vi "Initialize.vi"(8 "error in":errorcluster, 11 "Plugin in":refnum<class "DateTimeChannel.lvclass">) -> (0 "error out":errorcluster, 3 "Plugin out":refnum<class "DateTimeChannel.lvclass">)   [LabVIEW 2023, in "DateTimeChannel.lvlib" / "DateTimeChannel.lvclass"]
uses:
  DateTimeChannel.lvclass
  C:/Program Files/National Instruments/LabVIEW 2023/vi.lib/FlexLogger/SDK/PluginSDK.lvlibp/PEFClasses/SDK/Plugin/Plugin.lvclass
  <vilib>/FlexLogger/SDK/PluginSDK.lvlibp/PEFClasses/SDK/Processing Element/Timing Parameters.ctl
  <vilib>/FlexLogger/SDK/PluginSDK.lvlibp/PEFClasses/SDK/Processing Element/Timing Method.ctl
  <vilib>/FlexLogger/SDK/PluginSDK.lvlibp/PEFClasses/SDK/Channel/Data Type_v2.ctl
  <vilib>/FlexLogger/SDK/PluginSDK.lvlibp/PEFClasses/SDK/Producer Channel/Producer Channel.lvclass
  C:/Program Files/National Instruments/LabVIEW 2023/vi.lib/FlexLogger/SDK/PluginSDK.lvlibp/PEFClasses/SDK/Channel/Channel.lvclass
  Date Time Channel Global.vi
  <vilib>/FlexLogger/SDK/PluginSDK.lvlibp/PEFClasses/SDK/Plugin/ParameterAccess/Write String.vi
  <vilib>/FlexLogger/SDK/PluginSDK.lvlibp/PEFClasses/SDK/Producer Channel/Create Producer Channel_v2.vi
  <vilib>/FlexLogger/SDK/PluginSDK.lvlibp/PEFClasses/SDK/Plugin/Plugin.lvclass
  <vilib>/FlexLogger/SDK/PluginSDK.lvlibp/PEFClasses/SDK/Processing Element/Processing Element.lvclass
  C:/Program Files/National Instruments/LabVIEW 2023/vi.lib/FlexLogger/SDK/PluginSDK.lvlibp/PEFClasses/SDK/Processing Element/Processing Element.lvclass
  C:/dev/niflexlogger-plugins/plugins/DateTimeChannel/source/DateTimeChannel/DateTimeChannel.lvclass
  <vilib>/FlexLogger/SDK/PluginSDK.lvlibp
  <vilib>/FlexLogger/SDK/PluginSDK.lvlibp/PEFClasses/SDK/Channel/Channel.lvclass
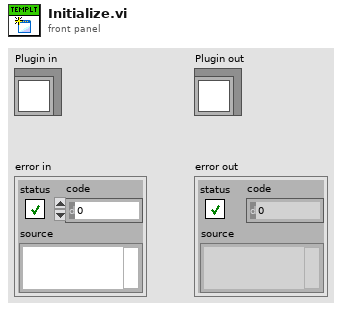
[diagram p1: front panel]
types:
  T1 = typedef "PluginSDK.lvlibp/Channel.lvclass/Data Type_v2.ctl" = u16
  T2 = typedef "PluginSDK.lvlibp/Processing Element.lvclass/Timing Parameters.ctl" = cluster{"Timing Method":T3, "Timing Period (ms)":i32}
  T3 = typedef "PluginSDK.lvlibp/Processing Element.lvclass/Timing Method.ctl" = enum16{"Periodic", "Immediate", "On Data Ready", "Triggered"}
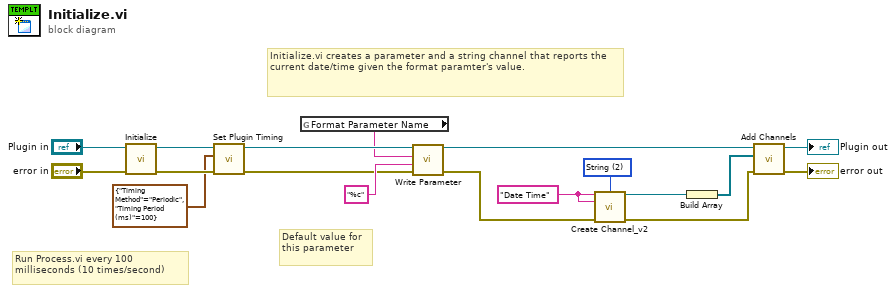
[diagram p0: block diagram]
diagram:
  w5 = "Date Time" ("Unique Channel Identifier")
  w6 = T1 2 items=["Wfm (DBL)", "Wfm (Digital)", "String"] ("Data Type")
  # "Default value for this parameter"
  # "Run Process.vi every 100 milliseconds (10 times/second)"
  # "Initialize.vi creates a parameter and a string channel that reports the current date/time given the format paramter's value."
  n1 = call-parent "Initialize.vi"("error in (no error)"="error in", "Plugin in"="Plugin in") -> ("error out"=w13:errorcluster, "Plugin out"=w11:refnum<class "DateTimeChannel.lvclass">)  [unwired: 8 in]
  n2 = call <vilib>:"Set Plugin Timing.vi"("error in (no error)"=w13, "Timing Parameters"=T2 {"Timing Method"=enum."Periodic", "Timing Period (ms)"=100}, "Plugin in"=w11) -> ("error out"=w9:errorcluster, "Plugin out"=w10:refnum<class "DateTimeChannel.lvclass">)  [unwired: 7 in]
  n3 = global read "Date Time Channel Global.vi" "Format Parameter Name"() -> (w1:string)
  n4 = call-poly <vilib>:"Write Parameter.vi"("error in (no error)"=w9, "Value"="%c", "Name"=w1, "Plugin in"=w10) -> ("error out"=w7:errorcluster, "Plugin out"=w8:refnum<class "DateTimeChannel.lvclass">)  [unwired: 6 in]
  n5 = call-poly <vilib>:"Create Channel_v2.vi"("Unique Channel Identifier"=w5, "Data Type"=w6, "Default Channel Name"=w5, "error in (no error)"=w7) -> ("Producer Channel"=w4:refnum<class "Producer Channel.lvclass">, "error out"=w2:errorcluster)  [unwired: 10 in]
  n6 = Build Array(w4) -> (w3:refnum<class "Producer Channel.lvclass">[])
  n7 = call <vilib>:"Add Channels.vi"("error in (no error)"=w2, "Channels"=w3, "Plugin in"=w8) -> ("error out"=→"error out":errorcluster, "Plugin out"=→"Plugin out":refnum<class "DateTimeChannel.lvclass">)  [unwired: 7 in]
